vi "ALR ACKs.vi"(8 "error in (no error)":errorcluster, 9 "Ack":bool, 10 "Index":i32[](array[numeric]), 11 "ALR_ON_OFF":T1) -> (0 "error out":errorcluster, 3 "ALR_ON_OFF out":T1)   [LabVIEW 2019, in "Alarms.lvlib"]
uses:
  Alarms.lvlib
  Ctl/ALR_ON_OFF.ctl
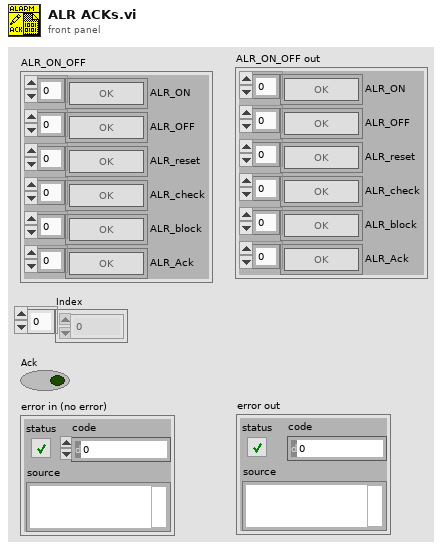
[diagram p1: front panel]
types:
  T1 = typedef "Alarms.lvlib/ALR_ON_OFF.ctl" = cluster{"ALR_ON":bool[], "ALR_OFF":bool[], "ALR_reset":bool[], "ALR_check":bool[], "ALR_block":bool[], "ALR_Ack":bool[]}
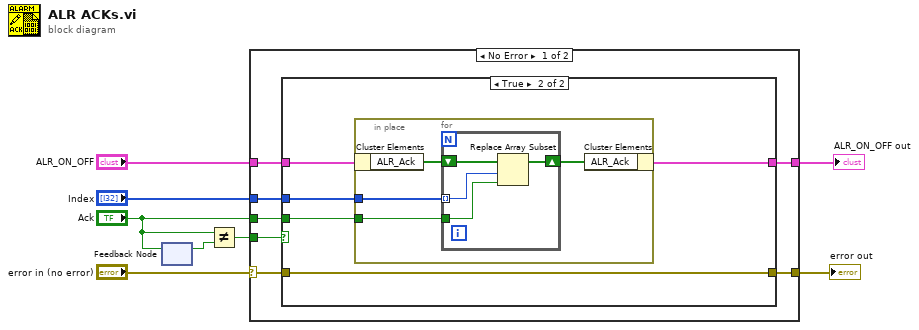
[diagram p0: block diagram]
diagram:
  n1 = feedback #1() -> (w5:bool)  [unwired: 1 in]
  n2 = feedback-in #1("Ack") -> ()
  n3 = Not Equal?(x="Ack", y=w5) -> (x != y?=w3:bool)
  n4 = case shown="No Error" "error in (no error)" {
    selector: "error in (no error)" -> [w11 w32]
    tunnel: "Index" -> [w15 _]
    tunnel: [w12 w32] -> w7
    tunnel: "ALR_ON_OFF" -> [w14 w31]
    tunnel: "Ack" -> [w13 _]
    tunnel: w3 -> [w10 _]
    tunnel: [w9 w31] -> w2
    frame No Error {
      n5 = case shown="True" w10 {
        tunnel: w15 -> [_ w22]
        tunnel: w14 -> [w16 w18]
        tunnel: w13 -> [_ w21]
        tunnel: [w17 w20] -> w12
        tunnel: w11 -> [w17 w20]
        tunnel: [w16 w19] -> w9
        frame False {
        }
        frame True {
          n6 = in-place {
            in-place-border: w22 -> [w25]
            in-place-border: w21 -> [w24]
            n7 = in-place-cluster #2(w18) -> ("ALR_Ack"=w26:bool[])
            n8 = for {
              tunnel: w25 -> [w29] mode=indexing
              tunnel: w24 -> [w28]
              shift-right: [w27] -> w23
              shift-left: w26 -> [w30]
              n9 = Replace Array Subset(array=w30, new element=w28, index=w29) -> (w27:bool[])
            }
            n10 = in-place-cluster #2("ALR_Ack"=w23) -> (w19:T1)
          }
        }
      }
    }
    frame Error {
    }
  }
  "error out" <- w7
  "ALR_ON_OFF out" <- w2
